vi "TCP-error.vi"   [LabVIEW 2013, in "SLMControl.lvlib" / "SM1000.lvclass"]
uses:
  SM1000.lvclass
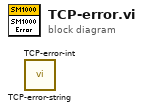
[diagram p0: block diagram]
diagram:
  n1 = call "TCP-error-string.vi"() -> ()  [unwired: 11 in, 1 out]
  n2 = call "TCP-error-int.vi"() -> ()  [unwired: 11 in, 1 out]
